vi "Sprinkler.vi"() -> ()   [LabVIEW 8.6]
doc: "This application simulates a sprinkler controller system that services four zones: North, South, East, and West. When simulaiton is started, the controller will proceed in order through the steps in the \"Zone Setup Array\". When the end of the array is reached, the controller will either stop (if \"Run Selector\" is set to Single, or will repeat the sequence from the start.\n\nWhen the application begins, intial values for the Zone Setup Array are loaded from a configuration file. This is a comma-separated text file which is named \"Sprinkler Configuration.txt\" and is expected to be in the root of the application directory.\n\nThe Setup button can be pressed at any time to enter Setup mode. While in setup mode, the simulation will stop and the Zone Setup array can be manually edited.\n\nPressing the \"Start\" button will begin simulation and will step throug the sequence defined in the Zone Setup Array. This array contains the desired zone as well as the duration for the current step. This array could be expanded for more information or more zones by modifying the type defs used in the project.\n\nWhile the simulation is running, the current zone and timing will be displayed in the \"Zone Indicators\".\n\nThe Simulator Controls can be used to set the water pressure of the system and control whether rain is detected. If water pressure is below 50% or rain is detected, the simulation will stop running. Once these conditions are removed, simulation will begin again from the first step of the sequence.\n\nNote: See \"Update Zone.vi\" documentation for description of behavior when Zone Array has invalid data (undefined zone or Timing of 0). U32 used instead of DBL for Timing to restrict user entry to positive integers (no decimal seconds)."
uses:
  Controls/State.ctl
  Controls/Zone Indicators.ctl
  Controls/Timer Actions.ctl
  Controls/Zone.ctl
  Controls/Zone Setup.ctl
panel:
  out "Controller Status":string
  in  "Simulation Controls":T1
  out "Zone Indicators":T2 {"Timing" format="%#.2g"}
  in  "Zone Setup Array":T3[](array[typedef])
  in  "Controls":T5
  # "Rain"
  # "No Rain"
  # "Continuous"
  # "Single"
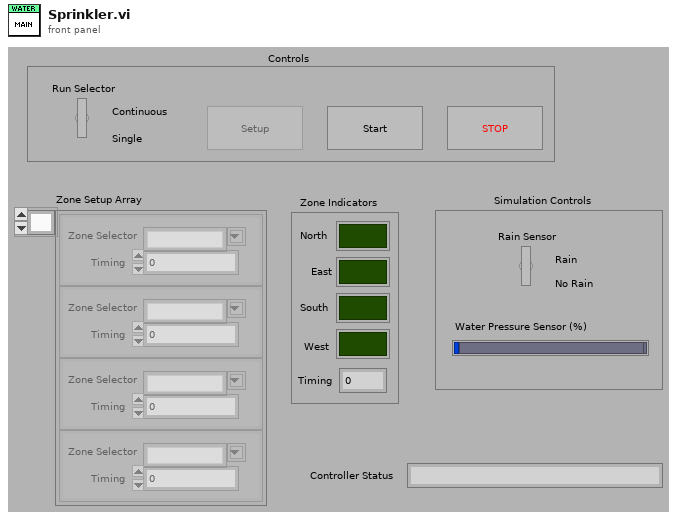
[diagram p1: front panel]
types:
  T1 = cluster{"Rain Sensor":bool, "Water Pressure Sensor (%)":dbl}
  T2 = typedef "Zone Indicators.ctl" = cluster{"North":bool, "East":bool, "South":bool, "West":bool, "Timing":dbl}
  T3 = typedef "Zone Setup.ctl" = cluster{"Zone Selector":T4, "Timing":u32}
  T4 = typedef "Zone.ctl" = string
  T5 = cluster{"Run Selector":bool, "Setup":bool, "Start":bool, "Stop":bool}
  T6 = typedef "State.ctl" = enum16{"Initialize", "Idle", "Setup", "Start", "Running", "Low Water Pressure", "Rain", "Stop"}
  T7 = enum8{"Enabled", "Disabled", "Disabled and Grayed Out"}
  T8 = typedef "Timer Actions.ctl" = enum16{"Reset", "Check Time"}
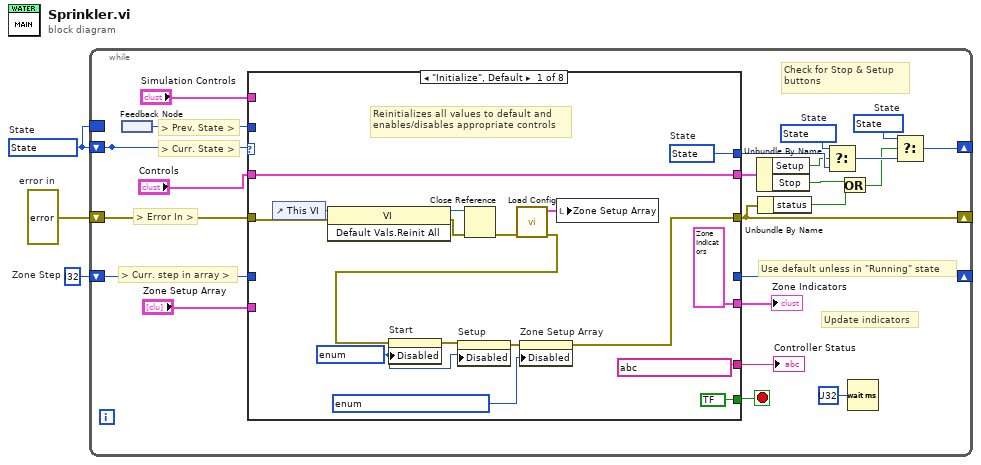
[diagram p0: block diagram]
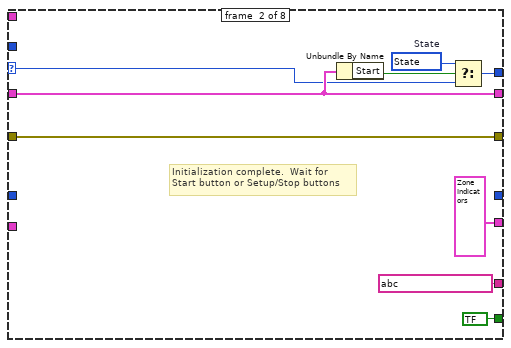
[diagram p2: hidden frame]
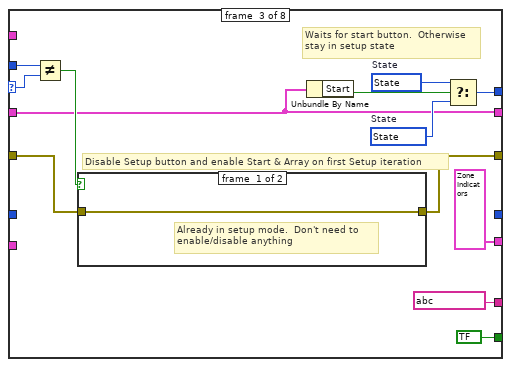
[diagram p3: hidden frame]
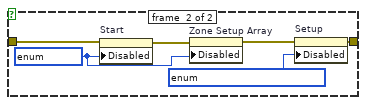
[diagram p4: hidden frame]
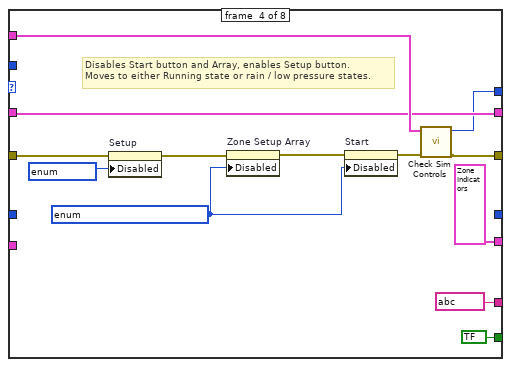
[diagram p5: hidden frame]
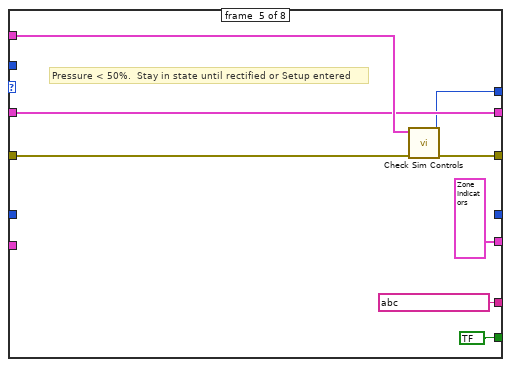
[diagram p6: hidden frame]
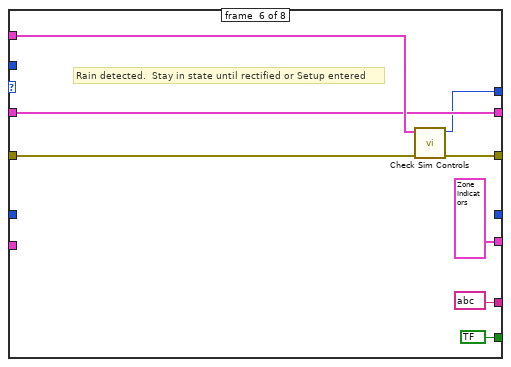
[diagram p7: hidden frame]
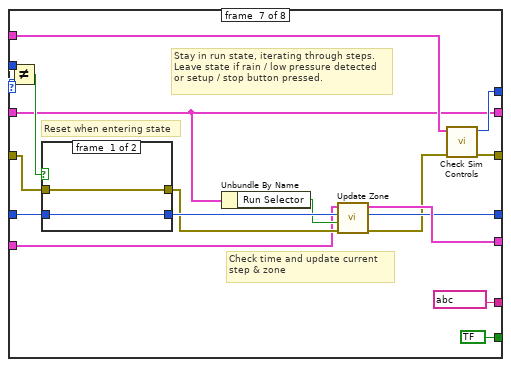
[diagram p8: hidden frame]
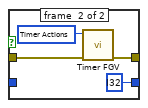
[diagram p9: hidden frame]
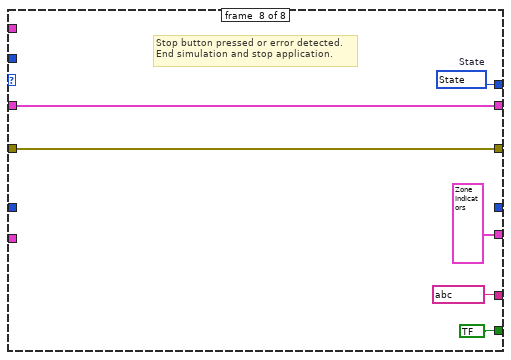
[diagram p10: hidden frame]
diagram:
  w1 = i32 ?  # Zone Step
  w3 = errorcluster ?  # error in
  w2 = T6 ?  # State
  n1 = while {
    shift-right: [w19] -> _
    shift-left: w2 -> [w18]
    shift-right: [w7] -> _
    shift-left: w3 -> [w22]
    border: w2 -> [_]
    shift-right: [w8] -> _
    shift-left: w1 -> [w10]
    stop <- w25 stop-if-true
    w14 = T6 ?  # State
    w15 = T6 ?  # State
    # "Use default unless in \"Running\" state"
    # "> Curr. step in array >"
    # "Update indicators"
    # "Check for Stop & Setup\nbuttons"
    # "> Error In >"
    # "> Curr. State >"
    # "> Prev. State >"
    n2 = feedback #1() -> (w17:T6)
    n3 = case shown="\"Initialize\", Default" w18 {
      selector: w18 -> [_ w45 w64 _ _ _ w115 _]
      tunnel: [bool ? bool ? bool ? bool ? bool ? bool ? bool ? bool ?] -> w25
      tunnel: [string ? string ? string ? string ? string ? string ? string ? string ?] -> w24
      tunnel: [T2 ? ("Zone Indicators") T2 ? ("Zone Indicators") T2 ? ("Zone Indicators") T2 ? ("Zone Indicators") T2 ? ("Zone Indicators") T2 ? ("Zone Indicators") w107 T2 ? ("Zone Indicators")] -> w23
      tunnel: w22 -> [w42 w47 w62 w76 w93 w101 w113 w128]
      tunnel: [w27 w47 w54 w77 w90 w98 w111 w128] -> w7
      tunnel: [w35 w50 w59 w81 w87 w95 w117 w126] -> w13
      tunnel: "Controls" -> [w34 w48 w57 w82 w89 w97 w109 w127]
      tunnel: [w34 w48 w57 w82 w89 w97 w109 w127] -> w20
      tunnel: w17 -> [_ _ w65 _ _ _ w116 _]
      tunnel: "Simulation Controls" -> [_ _ _ w85 w91 w99 w118 _]
      tunnel: w10 -> [_ _ _ _ _ _ w112 _]
      tunnel: "Zone Setup Array" -> [_ _ _ _ _ _ w103 _]
      tunnel: [_ _ _ _ _ _ w106 _] -> w8
      frame #0 {
        w29 = T7 ? ("Disabled")
        w35 = T6 ?  # State
        # "Reinitializes all values to default and \nenables/disables appropriate controls"
        n4 = control-ref of="This VI"() -> (w43:refnum<vi>)
        n5 = invoke class="VI" method="Default Vals.Reinit All"(reference=w43, error in=w42) -> (reference out=w40:refnum<vi>, error out=w41:errorcluster)  [unwired: 1 in, 1 out]
        n6 = Close Reference(reference=w40, error in (no error)=w41) -> (error out=w32:errorcluster)
        n7 = call "Load Config.vi"("error in"=w32) -> ("error out"=w31:errorcluster, "Zone Setup Array"=w33:T3[])  [unwired: 9 in]
        n8 = property on="Start" class="Bool"(error in=w31, "Disabled"=w29) -> (error out=w30:errorcluster)  [unwired: 1 in, 1 out]
        n9 = property on="Setup" class="Bool"(error in=w30, "Disabled"=w29) -> (error out=w28:errorcluster)  [unwired: 1 in, 1 out]
        n10 = property on="Zone Setup Array" class="Arr (strict)"(error in=w28, "Disabled"=T7 ?) -> (error out=w27:errorcluster)  [unwired: 1 in, 1 out]
        n11 = local write "Zone Setup Array"(w33) -> ()
      }
      frame #1 {
        w51 = T6 ?  # State
        # "Initialization complete.  Wait for\nStart button or Setup/Stop buttons"
        n12 = Unbundle By Name(w48) -> ("Start"=w52:bool)
        n13 = Select(t=w51, s=w52, f=w45) -> (s? t:f=w50:T6)
      }
      frame #2 {
        w58 = T6 ?  # State
        w60 = T6 ?  # State
        # "Waits for start button.  Otherwise\nstay in setup state"
        # "Disable Setup button and enable Start & Array on first Setup iteration"
        n14 = Not Equal?(x=w65, y=w64) -> (x != y?=w63:bool)
        n15 = case shown="True" w63 {
          tunnel: w62 -> [w66 w69]
          tunnel: [w66 w72] -> w54
          frame #0 {
            # "Already in setup mode.  Don't need to\nenable/disable anything"
          }
          frame #1 {
            w68 = T7 ? ("Disabled")
            n16 = property on="Start" class="Bool"(error in=w69, "Disabled"=w68) -> (error out=w67:errorcluster)  [unwired: 1 in, 1 out]
            n17 = property on="Zone Setup Array" class="Arr (strict)"(error in=w67, "Disabled"=w68) -> (error out=w71:errorcluster)  [unwired: 1 in, 1 out]
            n18 = property on="Setup" class="Bool"(error in=w71, "Disabled"=T7 ?) -> (error out=w72:errorcluster)  [unwired: 1 in, 1 out]
          }
        }
        n19 = Unbundle By Name(w57) -> ("Start"=w56:bool)
        n20 = Select(t=w60, s=w56, f=w58) -> (s? t:f=w59:T6)
      }
      frame #3 {
        w74 = T7 ? ("Disabled")
        # "Disables Start button and Array, enables Setup button.\nMoves to either Running state or rain / low pressure states."
        n21 = property on="Setup" class="Bool"(error in=w76, "Disabled"=T7 ?) -> (error out=w75:errorcluster)  [unwired: 1 in, 1 out]
        n22 = property on="Zone Setup Array" class="Arr (strict)"(error in=w75, "Disabled"=w74) -> (error out=w73:errorcluster)  [unwired: 1 in, 1 out]
        n23 = property on="Start" class="Bool"(error in=w73, "Disabled"=w74) -> (error out=w78:errorcluster)  [unwired: 1 in, 1 out]
        n24 = call "Check Sim Controls.vi"("error in (no error)"=w78, "Simulation Controls"=w85) -> ("error out"=w77:errorcluster, "State"=w81:T6)  [unwired: 8 in]
      }
      frame #4 {
        # "Pressure < 50%.  Stay in state until rectified or Setup entered"
        n25 = call "Check Sim Controls.vi"("error in (no error)"=w93, "Simulation Controls"=w91) -> ("error out"=w90:errorcluster, "State"=w87:T6)  [unwired: 8 in]
      }
      frame #5 {
        # "Rain detected.  Stay in state until rectified or Setup entered"
        n26 = call "Check Sim Controls.vi"("error in (no error)"=w101, "Simulation Controls"=w99) -> ("error out"=w98:errorcluster, "State"=w95:T6)  [unwired: 8 in]
      }
      frame #6 {
        # "Stay in run state, iterating through steps.\nLeave state if rain / low pressure detected\nor setup / stop button pressed."
        # "Check time and update current\nstep & zone"
        # "Reset when entering state"
        n27 = Not Equal?(x=w116, y=w115) -> (x != y?=w114:bool)
        n28 = case shown="True" w114 {
          tunnel: w113 -> [w121 w124]
          tunnel: [w121 w123] -> w104
          tunnel: w112 -> [w120 _]
          tunnel: [w120 i32 ? ("Zone Step")] -> w110
          frame #0 {
          }
          frame #1 {
            n29 = call "Timer FGV.vi"("error in"=w124, "Timer Action"=T8 ?) -> ("error out"=w123:errorcluster)  [unwired: 7 in, 2 out]
          }
        }
        n30 = Unbundle By Name(w109) -> ("Run Selector"=w108:bool)
        n31 = call "Update Zone.vi"("error in"=w104, "Run Selector"=w108, "Zone Step"=w110, "Zone Setup Array"=w103) -> ("error out"=w105:errorcluster, "Zone Step"=w106:i32, "Zone Indicators"=w107:T2)  [unwired: 5 in]
        n32 = call "Check Sim Controls.vi"("error in (no error)"=w105, "Simulation Controls"=w118) -> ("error out"=w111:errorcluster, "State"=w117:T6)  [unwired: 8 in]
      }
      frame #7 {
        w126 = T6 ?  # State
        # "Stop button pressed or error detected.\nEnd simulation and stop application."
      }
    }
    "Zone Indicators" <- w23
    "Controller Status" <- w24
    n33 = Unbundle By Name(w20) -> ("Setup"=w12:bool, "Stop"=w5:bool)
    n34 = Unbundle By Name(w7) -> ("status"=w6:bool)
    n35 = Select(t=w14, s=w12, f=w13) -> (s? t:f=w11:T6)
    n36 = Or(x=w5, y=w6) -> (x .or. y?=w4:bool)
    n37 = Wait (ms)(milliseconds to wait=u32 ?) -> ()  [unwired: 1 out]
    n38 = Select(t=w15, s=w4, f=w11) -> (s? t:f=w19:T6)
  }
